vi "Step Core.vi"(8 "error in (no error)":errorcluster, 11 "SPECAN_IQSLOT in":refnum<class "SPECAN_IQSLOT.lvclass">) -> (0 "error out":errorcluster, 3 "SPECAN_IQSLOT out":refnum<class "SPECAN_IQSLOT.lvclass">)   [LabVIEW 2018, in "SPECAN_IQSLOT.lvlib" / "SPECAN_IQSLOT.lvclass"]
uses:
  SPECAN_IQSLOT.lvclass
  Plugins/Measurement Interface.lvlibp/Measurement Interface.lvclass
  C:/Sequence Automation/Plugins/Measurement Interface.lvlibp/Measurement Interface.lvclass
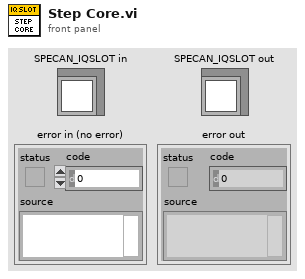
[diagram p1: front panel]
types:
  T1 = typedef "TestStand API Tools (TSAT).lvlibp/TSAT Evaluation Actions.lvlib/TSAT Evaluation.ctl" = cluster{"Test Name":string, "Pin":string, "Units":string, "SI Scaling":T2, "Test Number":i32, "Published Data Id":string, "Low Limit":dbl, "High Limit":dbl, "Export Data Location":string, "Software Bin":i64, "Evaluation Type":T3, "Test Data Source":string}
  T2 = typedef "TestStand API Tools (TSAT).lvlibp/TSAT Evaluation Actions.lvlib/TSAT Eval SI Unit Scaling.ctl" = i16
  T3 = typedef "TestStand API Tools (TSAT).lvlibp/TSAT Evaluation Actions.lvlib/TSAT Evaluation Type.ctl" = enum16{"Numeric Limit", "Pass/Fail", "None"}
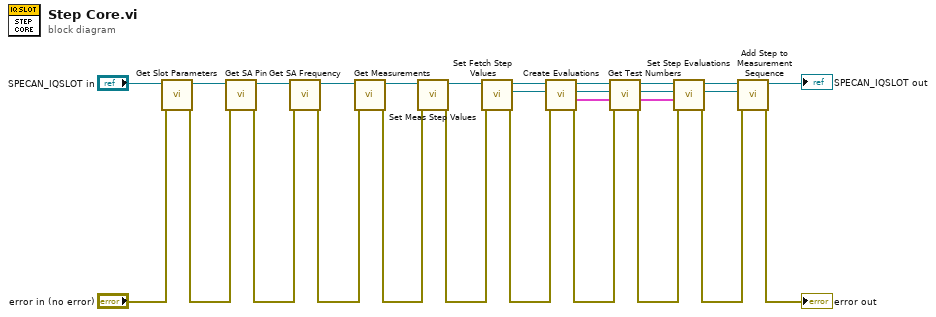
[diagram p0: block diagram]
diagram:
  n1 = call "Get Slot Parameters.vi"("error in (no error)"="error in (no error)", "SPECAN_IQSLOT in"="SPECAN_IQSLOT in") -> ("error out"=w3:errorcluster, "SPECAN_IQSLOT out"=w9:refnum<class "SPECAN_IQSLOT.lvclass">)  [unwired: 8 in]
  n2 = call-dynamic "Get SA Pin.vi"("error in (no error)"=w3, "SPECAN_IQSLOT in"=w9) -> ("error out"=w4:errorcluster, "SPECAN_IQSLOT out"=w8:refnum<class "SPECAN_IQSLOT.lvclass">)  [unwired: 8 in]
  n3 = call-dynamic "Get SA Frequency.vi"("error in (no error)"=w4, "SPECAN_IQSLOT in"=w8) -> ("error out"=w1:errorcluster, "SPECAN_IQSLOT out"=w7:refnum<class "SPECAN_IQSLOT.lvclass">)  [unwired: 8 in]
  n4 = call-dynamic "Get Measurements.vi"("error in (no error)"=w1, "SPECAN_IQSLOT in"=w7) -> ("error out"=w5:errorcluster, "SPECAN_IQSLOT out"=w6:refnum<class "SPECAN_IQSLOT.lvclass">)  [unwired: 8 in]
  n5 = call "Set Meas Step Values.vi"("error in (no error)"=w5, "SPECAN_IQSLOT in"=w6) -> ("error out"=w25:errorcluster, "SPECAN_IQSLOT out"=w26:refnum<class "SPECAN_IQSLOT.lvclass">)  [unwired: 8 in]
  n6 = call "Set Fetch Step Values.vi"("error in (no error)"=w25, "SPECAN_IQSLOT in"=w26) -> ("error out"=w21:errorcluster, "Step Out"=w20:refnum<k7>, "SPECAN_IQSLOT out"=w22:refnum<class "SPECAN_IQSLOT.lvclass">)  [unwired: 7 in]
  n7 = call-dynamic "Create Evaluations.vi"("error in (no error)"=w21, "SPECAN_IQSLOT in"=w22) -> ("error out"=w15:errorcluster, "Evaluations Out"=w12:T1[], "SPECAN_IQSLOT out"=w16:refnum<class "SPECAN_IQSLOT.lvclass">)  [unwired: 7 in]
  n8 = call "Get Test Numbers.vi"("error in (no error)"=w15, "Evaluations In"=w12, "SPECAN_IQSLOT in"=w16) -> ("error out"=w13:errorcluster, "Evaluations Out"=w11:T1[], "SPECAN_IQSLOT out"=w14:refnum<class "SPECAN_IQSLOT.lvclass">)  [unwired: 6 in]
  n9 = call-dynamic "Set Step Evaluations.vi"("error in (no error)"=w13, "Evaluation Data"=w11, "Step In"=w20, "SPECAN_IQSLOT in"=w14) -> ("error out"=w18:errorcluster, "Step out"=w17:refnum<k7>, "SPECAN_IQSLOT out"=w19:refnum<class "SPECAN_IQSLOT.lvclass">)  [unwired: 5 in]
  n10 = call "Add Step to Measurement Sequence.vi"("error in (no error)"=w18, "Step to Add"=w17, "Measurement Interface in"=w19) -> ("error out"=→"error out":errorcluster, "Measurement Interface out"=→"SPECAN_IQSLOT out":refnum<class "SPECAN_IQSLOT.lvclass">)  [unwired: 7 in]
